vi "API_LoadImages.vi"(6 "Timeout (ms)":u32, 7 "Wait (F)":bool, 8 "error in (no error)":errorcluster, 10 "LoadImagesData":T1, 11 "DLP2 in":refnum<class "DLP2.lvclass">) -> (0 "error out":errorcluster, 3 "DLP2 out":refnum<class "DLP2.lvclass">)   [LabVIEW 2022 SP3, in "DLP2.lvclass"]
doc: "Developed by Kevin Thompson\nkevin@thompsonengineering.net\n\nCopyright 2018\nThompson Engineering, LLC"
uses:
  DLP2.lvclass
  DataTypes/LoadImagesData--cluster.ctl
  DataTypes/AsynCmd_Temp01--enum.ctl
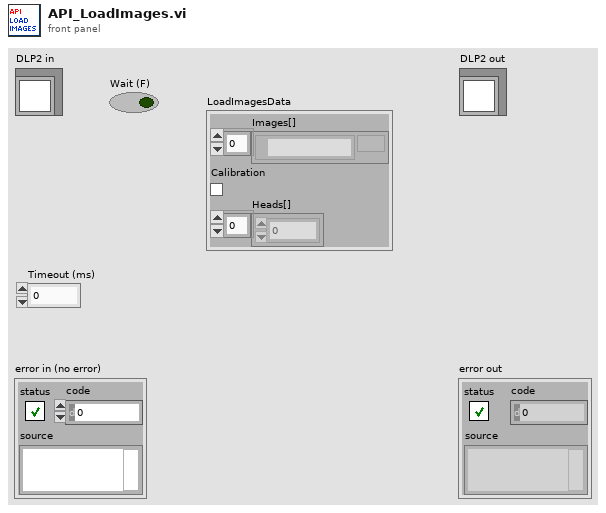
[diagram p1: front panel]
types:
  T1 = typedef "LoadImagesData--cluster.ctl" = cluster{"Images[]":path[], "Calibration":bool, "Heads[]":u8[]}
  T2 = typedef "DLP2.lvclass/AsynCmd_Temp01--enum.ctl" = enum16{"LoadTiffImage", "SeperateLayersPython", "InvokePPP", "LoadImages"}
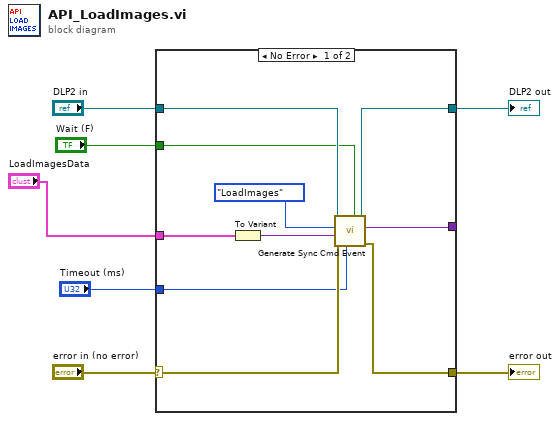
[diagram p0: block diagram]
diagram:
  n1 = case shown="No Error" "error in (no error)" {
    selector: "error in (no error)" -> [w15 w19]
    tunnel: [w9 w19] -> w6
    tunnel: [w16 w18] -> w4
    tunnel: "DLP2 in" -> [w17 w18]
    tunnel: "LoadImagesData" -> [w13 _]
    tunnel: "Wait (F)" -> [w11 _]
    tunnel: "Timeout (ms)" -> [w10 _]
    tunnel: [w8 _] -> _
    frame No Error {
      n2 = To Variant(anything=w13) -> (Variant=w12:variant)
      n3 = call "Generate Sync Cmd Event.vi"("Wait (F)"=w11, "Timeout (ms)"=w10, "error in (no error)"=w15, "vData"=w12, "AsyncCmd"=AsynCmd_Temp01--enum."LoadImages", "DLP2 in"=w17) -> ("error out"=w9:errorcluster, "Return Value"=w8:variant, "DLP2 out"=w16:refnum<class "DLP2.lvclass">)  [unwired: 3 in]
    }
    frame Error {
    }
  }
  "error out" <- w6
  "DLP2 out" <- w4
